vi "Teleop.vi"(10 "Match Info":T1={"Autonomous Elapsed Seconds"=0.0, "TeleOp Elapsed Seconds"=0.0, "Disabled Elapsed Seconds"=0.0, "Visited Autonomous"=FALSE, "Visited TeleOp"=FALSE, "Visited Disabled"=FALSE, "Autonomous Settings"={"Autonomous Style"=enum."Independent", "VI Refnum"=refnum}}, 11 "Call Context":T2) -> ()   [LabVIEW 2015]
doc: "This VI is called for each enabled TeleOp packet received from the DS. It is typically used to read from joysticks and other inputs and update I/O or setpoints for timed control loops. It should complete and return within 20 milliseconds or risk missing DS packets."
uses:
  <vilib>/Rock Robotics/WPI/DriverStation/WPI_DriverStationDerivedRobotMode.ctl
  <vilib>/Rock Robotics/WPI/DriverStation/WPI_DriverStationMatch Info.ctl
  AutoTask SubVI/TeleopDrive.ctl
  <vilib>/Rock Robotics/WPI/Solenoid/WPI_SolenoidValue.ctl
  AutoTask/Implementation/AutoTask Setpoints.ctl
  AutoTask/Implementation/AutoTask Operations.ctl
  <vilib>/Rock Robotics/WPI/Utilities/WPI_GetSetVariantRefNum.vi
  <vilib>/Rock Robotics/Network Tables/NT Write Boolean Array.vi
  <vilib>/Rock Robotics/Network Tables/NT Write Numeric Array.vi
  <vilib>/Rock Robotics/WPI/Solenoid/WPI_SolenoidSetEnum.vi
  <vilib>/Rock Robotics/Network Tables/NT Read Number.vi
  Framework/Robot Global Data.vi
  NavX/navX Library v2/navX Library v2.lvlib
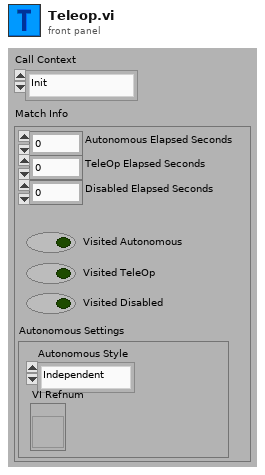
[diagram p1: front panel]
types:
  T1 = typedef "WPI_DriverStationMatch Info.ctl" = cluster{"Autonomous Elapsed Seconds":dbl, "TeleOp Elapsed Seconds":dbl, "Disabled Elapsed Seconds":dbl, "Visited Autonomous":bool, "Visited TeleOp":bool, "Visited Disabled":bool, "Autonomous Settings":cluster{"Autonomous Style":enum16{"Iterative", "Independent"}, "VI Refnum":refnum<vi>}}
  T2 = typedef "WPI_DriverStationDerivedRobotMode.ctl" = enum16{"Init", "Execute", "Stop"}
  T3 = typedef "TeleopDrive.ctl" = enum16{"Joystick", "AutoTurn", "AutoAlign", "GearShifter", "Stop", "DriveDistance", "LiftPneuDown", "LiftPneuUp", "CatA OpenUp", "CatA OpenDown", "Intake", "AutoIntake", "AutoOuttake"}
  T4 = typedef "WPI_JoystickDevRef.ctl" = cluster{"Device":T5}
  T5 = typedef "WPI_JoystickDeviceEnum.ctl" = enum16{"USB 0", "USB 1", "USB 2", "USB 3", "USB 4", "USB 5"}
  T6 = typedef "WPI_SolenoidValue.ctl" = enum16{"Off", "On", "Forward", "Reverse"}
  T7 = typedef "WPI_SolenoidDevRef.ctl" = cluster{"DevStatus":errorcluster, "Pneumatics Control Module":u8, "Forward Solenoid Channel":T8, "Reverse Solenoid Channel":T8}
  T8 = typedef "WPI_SolenoidChannel.ctl" = enum8{"Solenoid 0", "Solenoid 1", "Solenoid 2", "Solenoid 3", "Solenoid 4", "Solenoid 5", "Solenoid 6", "Solenoid 7", "Invalid"}
  T9 = typedef "AutoTask Setpoints.ctl" = cluster{"Operation":T10, "Setpoint":dbl, "Duration":dbl, "Speed":dbl, "Angle":dbl, "VDeadband":dbl, "Deadband":dbl}
  T10 = typedef "AutoTask Operations.ctl" = enum16{"Reserve", "Read Current", "Immediate", "DriveDistance", "AutoShoot", "FaceForward", "AutoAlign", "AutoTurn", "DriveToLine", "DriveToIncline", "DriveTillFlat"}
  T11 = typedef "navX Library v2.lvlib/Z900_navX_DeviceTypeDef.ctl" = cluster{"Interface":cluster{"Protocol":T12, "Update Rate (4Hz-60Hz)":u8, "navX Open TypeDef":variant}, "Notify Packet":refnum<notifier>, "Loop VI Refnum":refnum<vi>, "Ready to Close Occurrence Refnum":refnum<k4>}
  T12 = typedef "navX Library v2.lvlib/Z900_navX_ProtocolTypeDef.ctl" = enum16{"SERIAL", "I2C", "SPI"}
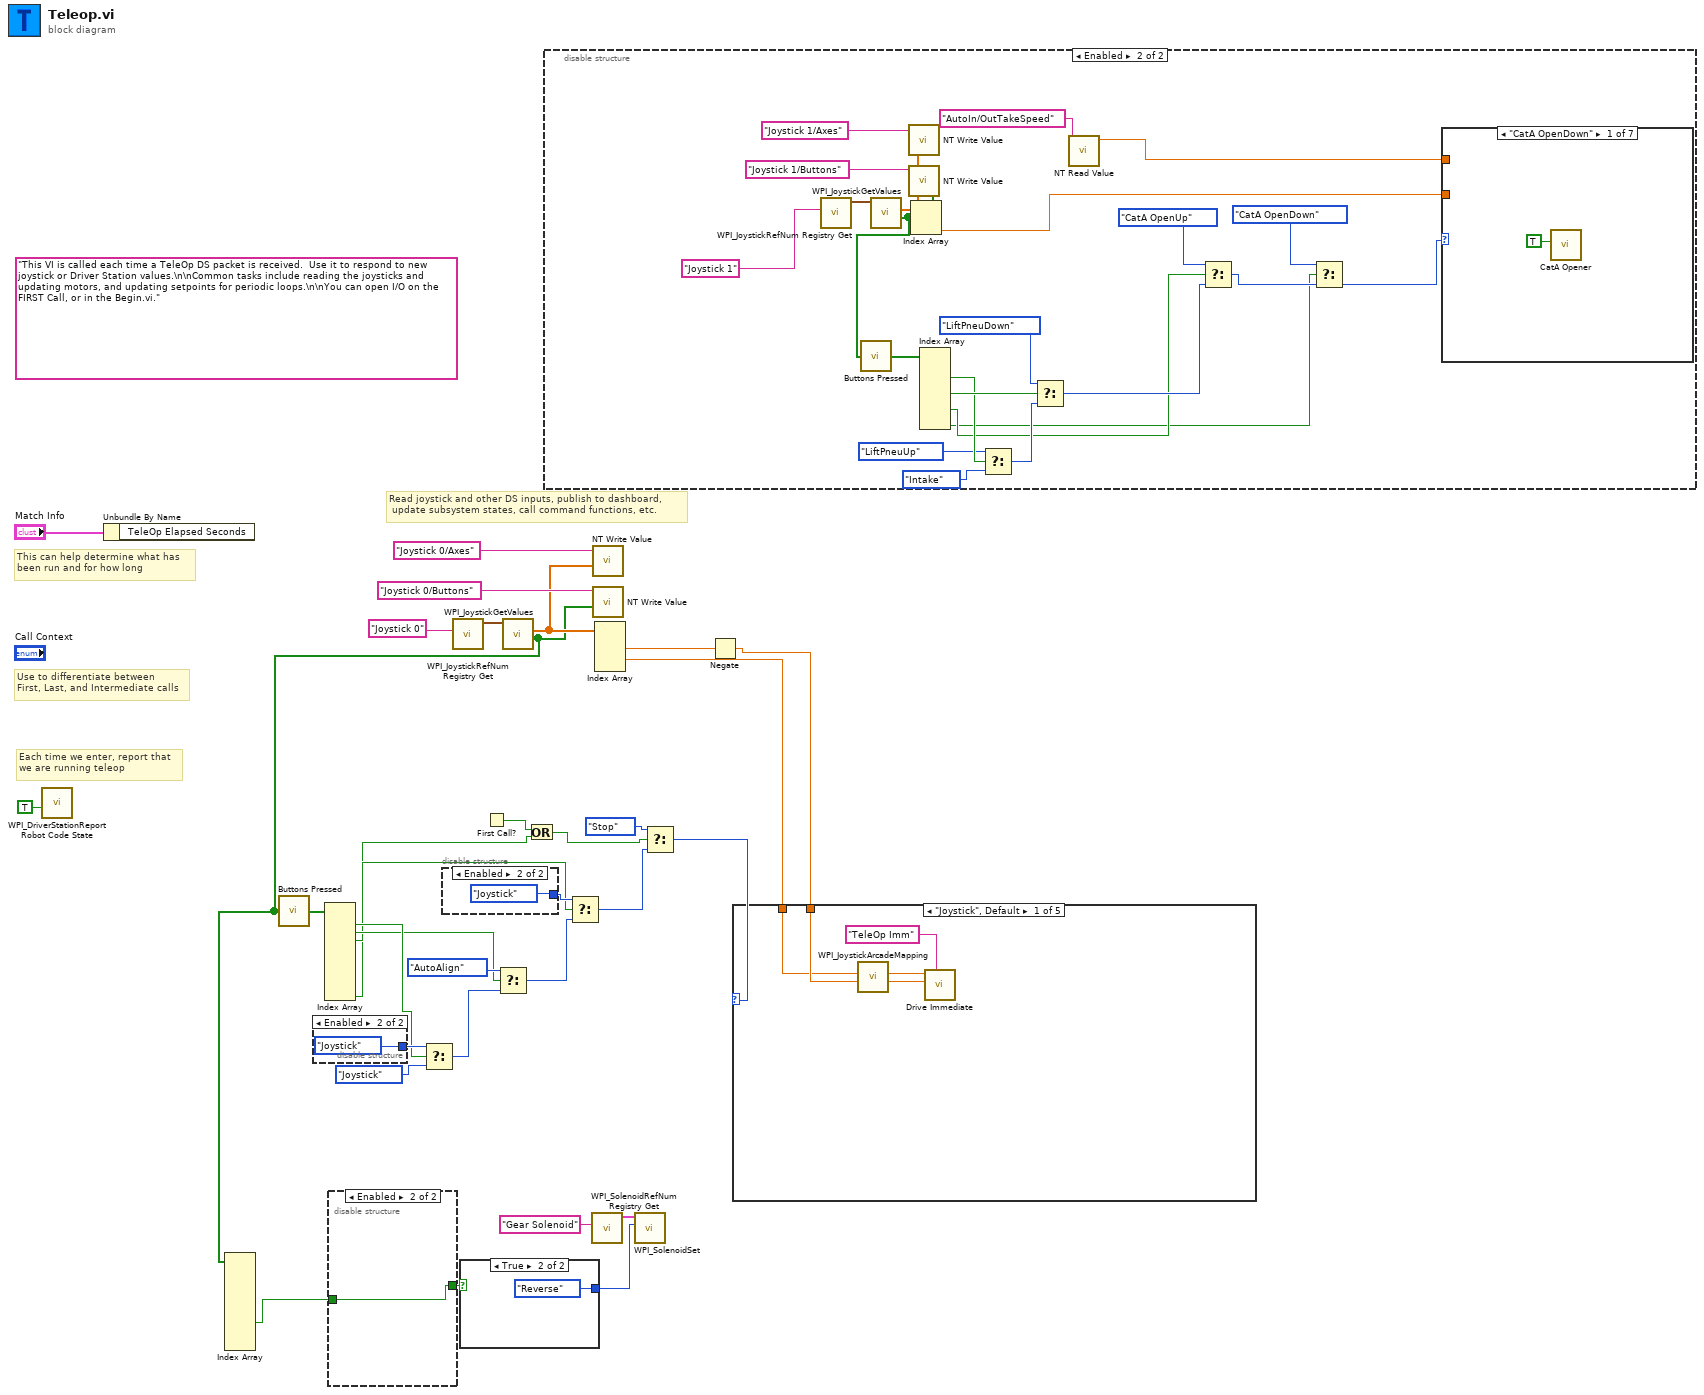
[diagram p0: block diagram]
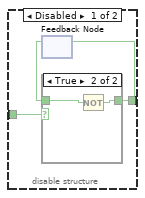
[diagram p2: hidden frame]
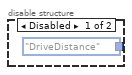
[diagram p4: hidden frame]
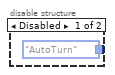
[diagram p5: hidden frame]
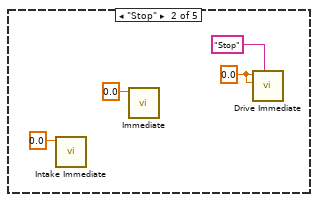
[diagram p6: hidden frame]
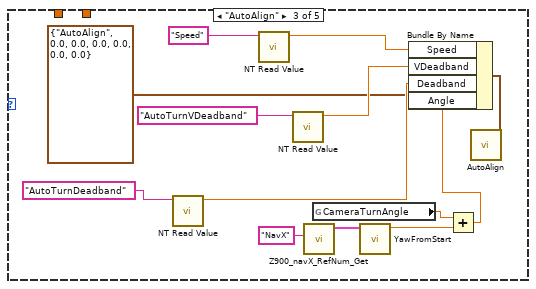
[diagram p7: hidden frame]
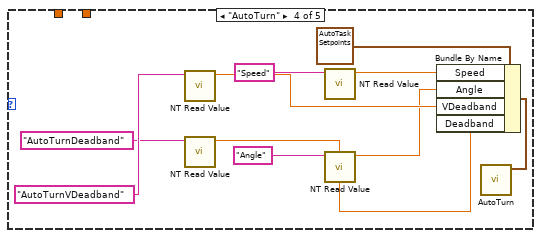
[diagram p8: hidden frame]
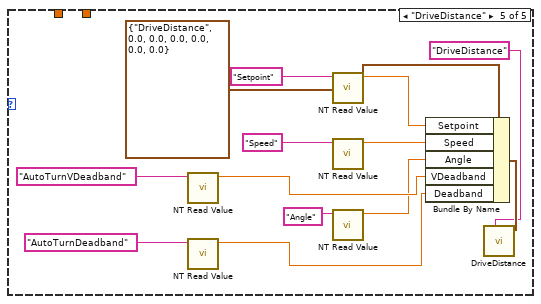
[diagram p9: hidden frame]
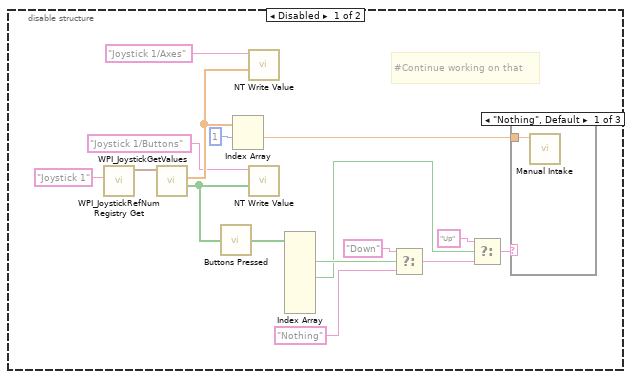
[diagram p10: hidden frame]
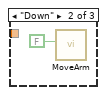
[diagram p11: hidden frame]
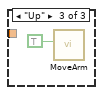
[diagram p12: hidden frame]
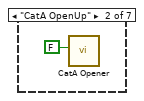
[diagram p13: hidden frame]
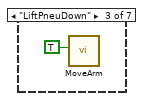
[diagram p14: hidden frame]
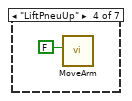
[diagram p15: hidden frame]
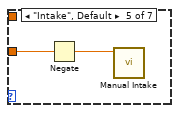
[diagram p16: hidden frame]
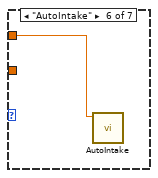
[diagram p17: hidden frame]
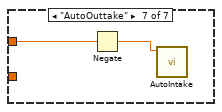
[diagram p18: hidden frame]
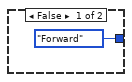
[diagram p19: hidden frame]
diagram:
  (unwired) "This VI is called each time a TeleOp DS packet is received.  Use it to respond to new joystick or Driver Station values.\n\nCommon tasks include reading the joysticks and updating motors, and updating setpoints for periodic loops.\n\nYou can open I/O on the FIRST Call, or in the Begin.vi."
  # "Read joystick and other DS inputs, publish to dashboard,\n update subsystem states, call command functions, etc."
  # "Each time we enter, report that\nwe are running teleop"
  # "Use to differentiate between\nFirst, Last, and Intermediate calls"
  # "This can help determine what has\nbeen run and for how long"
  n1 = call <vilib>:"WPI_DriverStationReport Robot Code State.vi"("TeleOp"=TRUE ("Autonomous")) -> ()  [unwired: 10 in, 1 out]
  n2 = Unbundle By Name("Match Info") -> ()  [unwired: 1 out]
  n3 = disable-structure shown="Enabled" {
    disable-tunnel: [TeleopDrive."AutoTurn" ("Enum") TeleopDrive."Joystick" ("Enum")] -> w23
    frame Disabled {
    }
    frame Enabled {
    }
  }
  n4 = disable-structure shown="Enabled" {
    disable-tunnel: [TeleopDrive."DriveDistance" ("Enum") TeleopDrive."Joystick" ("Enum")] -> w17
    frame Disabled {
    }
    frame Enabled {
    }
  }
  n5 = call <vilib>:"WPI_JoystickRefNum Registry Get.vi"("refnum name"="Joystick 0") -> ("JoystickDevRef"=w29:T4)  [unwired: 1 in, 9 out]
  n6 = First Call?() -> (First Call?: T/F=w1:bool)
  n7 = call <vilib>:"WPI_JoystickGetValues.vi"("JoystickDevRef"=w29) -> ("Buttons"=w5:bool[], "Axes"=w27:dbl[])  [unwired: 6 in, 3 out]
  n8 = Index Array(array=w5) -> (element #7=w4:bool)  [unwired: 10 in, 9 out]
  n9 = call "Buttons Pressed.vi"("Button Values"=w5) -> ("Button Presses"=w25:bool[])
  n10 = Index Array(array=w25) -> (element #1=w22:bool, element #2=w19:bool, element #3=w16:bool, element #10=w3:bool)  [unwired: 10 in, 6 out]
  n11 = disable-structure shown="Enabled" {
    disable-tunnel: w4 -> [w38 w43]
    disable-tunnel: [w37 w43] -> w9
    frame Disabled {
      n12 = feedback #1() -> (w39:bool)  [unwired: 1 in]
      n13 = case shown="True" w38 {
        tunnel: [w40 w42] -> w37
        tunnel: w39 -> [w40 w41]
        frame False {
        }
        frame True {
          n14 = Not(x=w41) -> (.not. x?=w42:bool)
        }
      }
      n15 = feedback-in #1(w37) -> ()
    }
    frame Enabled {
    }
  }
  n16 = Select(t=w23, s=w22, f=TeleopDrive."Joystick" ("Enum")) -> (s? t:f=w21:T3)
  n17 = case shown="True" w9 {
    tunnel: [WPI_SolenoidValue."Forward" ("Value") WPI_SolenoidValue."Reverse" ("Value")] -> w8
    frame False {
    }
    frame True {
    }
  }
  n18 = Select(t=TeleopDrive."AutoAlign" ("Enum"), s=w19, f=w21) -> (s? t:f=w18:T3)
  n19 = Or(x=w1, y=w3) -> (x .or. y?=w2:bool)
  n20 = disable-structure shown="Enabled" {
    frame Disabled {
      # "#Continue working on that"
      n21 = call <vilib>:"WPI_JoystickRefNum Registry Get.vi"("refnum name"="Joystick 1") -> ("JoystickDevRef"=w54:T4)  [unwired: 1 in, 9 out]
      n22 = call <vilib>:"WPI_JoystickGetValues.vi"("JoystickDevRef"=w54) -> ("Buttons"=w56:bool[], "Axes"=w55:dbl[])  [unwired: 6 in, 3 out]
      n23 = call "Buttons Pressed.vi"("Button Values"=w56) -> ("Button Presses"=w57:bool[])
      n24 = Index Array(array=w55, index #1=1 ("index")) -> (element #1=w46:dbl)  [unwired: 1 in, 1 out]
      n25 = call-poly <vilib>:"NT Write Value.vi"("Numeric Array"=w55, "Name"="Joystick 1/Axes") -> ()  [unwired: 9 in, 1 out]
      n26 = call-poly <vilib>:"NT Write Value.vi"("Boolean Array"=w56, "Name"="Joystick 1/Buttons") -> ()  [unwired: 9 in, 1 out]
      n27 = Index Array(array=w57) -> (element #2=w59:bool, element #4=w58:bool)  [unwired: 8 in, 6 out]
      n28 = Select(t="Down", s=w59, f="Nothing") -> (s? t:f=w60:string)
      n29 = Select(t="Up", s=w58, f=w60) -> (s? t:f=w61:string)
      n30 = case shown="\"Nothing\", Default" w61 {
        tunnel: w46 -> [w62 _ _]
        frame "Nothing", Default {
          n31 = call "Manual Intake.vi"("Setpoint"=w62) -> ()  [unwired: 10 in, 1 out]
        }
        frame "Down" {
          n32 = call "MoveArm.vi"("OnOff"=FALSE) -> ()  [unwired: 10 in, 1 out]
        }
        frame "Up" {
          n33 = call "MoveArm.vi"("OnOff"=TRUE) -> ()  [unwired: 10 in, 1 out]
        }
      }
    }
    frame Enabled {
      n34 = call <vilib>:"WPI_JoystickRefNum Registry Get.vi"("refnum name"="Joystick 1") -> ("JoystickDevRef"=w74:T4)  [unwired: 1 in, 9 out]
      n35 = call <vilib>:"WPI_JoystickGetValues.vi"("JoystickDevRef"=w74) -> ("Buttons"=w77:bool[], "Axes"=w72:dbl[])  [unwired: 6 in, 3 out]
      n36 = call "Buttons Pressed.vi"("Button Values"=w77) -> ("Button Presses"=w76:bool[])
      n37 = call-poly <vilib>:"NT Write Value.vi"("Numeric Array"=w72, "Name"="Joystick 1/Axes") -> ()  [unwired: 9 in, 1 out]
      n38 = call-poly <vilib>:"NT Write Value.vi"("Boolean Array"=w77, "Name"="Joystick 1/Buttons") -> ()  [unwired: 9 in, 1 out]
      n39 = Index Array(array=w72) -> (element #2=w84:dbl)  [unwired: 2 in, 1 out]
      n40 = Index Array(array=w76) -> (element #2=w80:bool, element #4=w82:bool, element #6=w66:bool, element #8=w65:bool)  [unwired: 8 in, 4 out]
      n41 = Select(t=TeleopDrive."LiftPneuUp" ("Enum"), s=w80, f=TeleopDrive."Intake" ("Enum")) -> (s? t:f=w81:T3)
      n42 = Select(t=TeleopDrive."LiftPneuDown" ("Enum"), s=w82, f=w81) -> (s? t:f=w85:T3)
      n43 = call-poly <vilib>:"NT Read Value.vi"("Name"="AutoIn/OutTakeSpeed") -> ("Numeric"=w87:dbl)  [unwired: 9 in, 1 out]
      n44 = Select(t=TeleopDrive."CatA OpenUp" ("Enum"), s=w66, f=w85) -> (s? t:f=w70:T3)
      n45 = Select(t=TeleopDrive."CatA OpenDown" ("Enum"), s=w65, f=w70) -> (s? t:f=w68:T3)
      n46 = case shown="\"CatA OpenDown\"" w68 {
        tunnel: w84 -> [_ _ _ _ w93 _ _]
        tunnel: w87 -> [_ _ _ _ _ w94 w96]
        frame "CatA OpenDown" {
          n47 = call "CatA Opener.vi"("OnOff"=TRUE) -> ()  [unwired: 10 in, 1 out]
        }
        frame "CatA OpenUp" {
          n48 = call "CatA Opener.vi"("OnOff"=FALSE) -> ()  [unwired: 10 in, 1 out]
        }
        frame "LiftPneuDown" {
          n49 = call "MoveArm.vi"("OnOff"=TRUE) -> ()  [unwired: 10 in, 1 out]
        }
        frame "LiftPneuUp" {
          n50 = call "MoveArm.vi"("OnOff"=FALSE) -> ()  [unwired: 10 in, 1 out]
        }
        frame "Intake", Default {
          n51 = Negate(x=w93) -> (-x=w92:dbl)
          n52 = call "Manual Intake.vi"("Setpoint"=w92) -> ()  [unwired: 10 in, 1 out]
        }
        frame "AutoIntake" {
          n53 = call "AutoIntake.vi"("Setpoint"=w94) -> ()  [unwired: 10 in, 1 out]
        }
        frame "AutoOuttake" {
          n54 = Negate(x=w96) -> (-x=w95:dbl)
          n55 = call "AutoIntake.vi"("Setpoint"=w95) -> ()  [unwired: 10 in, 1 out]
        }
      }
    }
  }
  n56 = Select(t=w17, s=w16, f=w18) -> (s? t:f=w11:T3)
  n57 = call <vilib>:"WPI_SolenoidRefNum Registry Get.vi"("refnum name"="Gear Solenoid") -> ("SolenoidDevRef"=w12:T7)  [unwired: 9 in, 1 out]
  n58 = call-poly <vilib>:"NT Write Value.vi"("Numeric Array"=w27, "Name"="Joystick 0/Axes") -> ()  [unwired: 9 in, 1 out]
  n59 = call-poly <vilib>:"NT Write Value.vi"("Boolean Array"=w5, "Name"="Joystick 0/Buttons") -> ()  [unwired: 9 in, 1 out]
  n60 = Index Array(array=w27) -> (element #2=w6:dbl, element #3=w10:dbl)  [unwired: 4 in, 2 out]
  n61 = call-poly <vilib>:"WPI_SolenoidSet.vi"("Value"=w8, "SolenoidDevRef"=w12) -> ()  [unwired: 8 in, 2 out]
  n62 = Select(t=TeleopDrive."Stop" ("Enum"), s=w2, f=w11) -> (s? t:f=w14:T3)
  n63 = Negate(x=w6) -> (-x=w7:dbl)
  n64 = case shown="\"Joystick\", Default" w14 {
    tunnel: w7 -> [w98 _ _ _ _]
    tunnel: w10 -> [w97 _ _ _ _]
    frame "Joystick", Default {
      n65 = call <vilib>:"WPI_JoystickArcadeMapping.vi"("Y axis value"=w98, "X axis value"=w97) -> ("Right Motor Value"=w101:dbl, "Left Motor Value"=w100:dbl)  [unwired: 8 in]
      n66 = call "Drive Immediate.vi"("Description"="TeleOp Imm", "Right Setpoint"=w101, "Left Setpoint"=w100) -> ()  [unwired: 8 in, 1 out]
    }
    frame "Stop" {
      w104 = 0.0
      n67 = call "Intake Immediate.vi"("Setpoint"=0.0) -> ()  [unwired: 10 in, 1 out]
      n68 = call "Immediate.vi"("Setpoint"=0.0) -> ()  [unwired: 10 in, 1 out]
      n69 = call "Drive Immediate.vi"("Description"="Stop", "Right Setpoint"=w104, "Left Setpoint"=w104) -> ()  [unwired: 8 in, 1 out]
    }
    frame "AutoAlign" {
      n70 = call-poly <vilib>:"NT Read Value.vi"("Name"="AutoTurnDeadband") -> ("Numeric"=w111:dbl)  [unwired: 9 in, 1 out]
      n71 = call-poly <vilib>:"NT Read Value.vi"("Name"="Speed") -> ("Numeric"=w113:dbl)  [unwired: 9 in, 1 out]
      n72 = call-poly <vilib>:"NT Read Value.vi"("Name"="AutoTurnVDeadband") -> ("Numeric"=w109:dbl)  [unwired: 9 in, 1 out]
      n73 = call "Z900_navX_RefNum_Get.vi"("refnum name"="NavX") -> ("navX Device"=w116:T11)  [unwired: 9 in, 1 out]
      n74 = global read "Robot Global Data.vi" "CameraTurnAngle"() -> (w114:dbl)
      n75 = call "YawFromStart.vi"("navX Device"=w116) -> ("Yaw"=w117:dbl)  [unwired: 10 in]
      n76 = Add(x=w114, y=w117) -> (x+y=w118:dbl)
      n77 = Bundle By Name(cluster=T9 {"Operation"=enum."AutoAlign", "Setpoint"=0.0, "Duration"=0.0, "Speed"=0.0, "Angle"=0.0, "VDeadband"=0.0, "Deadband"=0.0} ("SubSystem Data"), "Speed"=w113, "VDeadband"=w109, "Deadband"=w111, "Angle"=w118) -> (w106:T9)
      n78 = call "AutoAlign.vi"("SubSystem Data"=w106) -> ()  [unwired: 10 in, 1 out]
    }
    frame "AutoTurn" {
      n79 = call-poly <vilib>:"NT Read Value.vi"("Name"="AutoTurnVDeadband") -> ("Numeric"=w127:dbl)  [unwired: 9 in, 1 out]
      n80 = call-poly <vilib>:"NT Read Value.vi"("Name"="AutoTurnDeadband") -> ("Numeric"=w125:dbl)  [unwired: 9 in, 1 out]
      n81 = call-poly <vilib>:"NT Read Value.vi"("Name"="Speed") -> ("Numeric"=w121:dbl)  [unwired: 9 in, 1 out]
      n82 = call-poly <vilib>:"NT Read Value.vi"("Name"="Angle") -> ("Numeric"=w123:dbl)  [unwired: 9 in, 1 out]
      n83 = Bundle By Name(cluster=T9 {"Operation"=enum."AutoTurn", "Setpoint"=0.0, "Duration"=0.0, "Speed"=0.0, "Angle"=0.0, "VDeadband"=0.0, "Deadband"=0.0} ("SubSystem Data"), "Speed"=w121, "Angle"=w123, "VDeadband"=w127, "Deadband"=w125) -> (w128:T9)
      n84 = call "AutoTurn.vi"("SubSystem Data"=w128) -> ()  [unwired: 9 in, 1 out]
    }
    frame "DriveDistance" {
      n85 = call-poly <vilib>:"NT Read Value.vi"("Name"="AutoTurnVDeadband") -> ("Numeric"=w140:dbl)  [unwired: 9 in, 1 out]
      n86 = call-poly <vilib>:"NT Read Value.vi"("Name"="AutoTurnDeadband") -> ("Numeric"=w136:dbl)  [unwired: 9 in, 1 out]
      n87 = call-poly <vilib>:"NT Read Value.vi"("Name"="Setpoint") -> ("Numeric"=w138:dbl)  [unwired: 9 in, 1 out]
      n88 = call-poly <vilib>:"NT Read Value.vi"("Name"="Speed") -> ("Numeric"=w132:dbl)  [unwired: 9 in, 1 out]
      n89 = call-poly <vilib>:"NT Read Value.vi"("Name"="Angle") -> ("Numeric"=w134:dbl)  [unwired: 9 in, 1 out]
      n90 = Bundle By Name(cluster=T9 {"Operation"=enum."DriveDistance", "Setpoint"=0.0, "Duration"=0.0, "Speed"=0.0, "Angle"=0.0, "VDeadband"=0.0, "Deadband"=0.0} ("SubSystem Data"), "Setpoint"=w138, "Speed"=w132, "Angle"=w134, "VDeadband"=w140, "Deadband"=w136) -> (w141:T9)
      n91 = call "DriveDistance.vi"("Description"="DriveDistance", "SubSystem Data"=w141) -> ()  [unwired: 9 in, 1 out]
    }
  }
